vi "Pusher_Client_PingPong.vi"(8 "ErrIn":errorcluster, 11 "Client in":refnum<class "Client.lvclass">) -> (0 "ErrOut":errorcluster, 3 "Client out":refnum<class "Client.lvclass">)   [LabVIEW 2009, in "Client.lvclass"]
uses:
  Client.lvclass
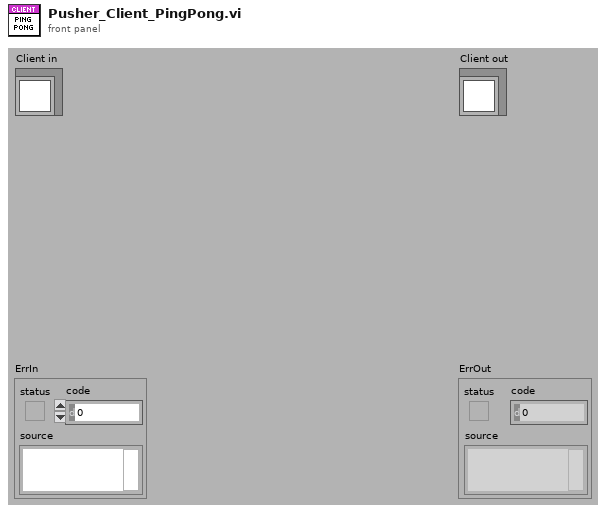
[diagram p1: front panel]
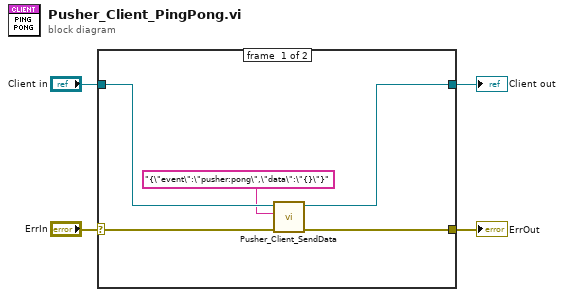
[diagram p0: block diagram]
diagram:
  n1 = case shown="No Error" "ErrIn" {
    selector: "ErrIn" -> [w9 w11]
    tunnel: [w8 w11] -> w3
    tunnel: [w6 w10] -> w1
    tunnel: "Client in" -> [w7 w10]
    frame #0 {
      n2 = call "Pusher_Client_SendData.vi"("ErrIn"=w9, "data"="{\"event\":\"pusher:pong\",\"data\":\"{}\"}", "Client in"=w7) -> ("ErrOut"=w8:errorcluster, "Client out"=w6:refnum<class "Client.lvclass">)  [unwired: 7 in]
    }
    frame #1 {
    }
  }
  "ErrOut" <- w3
  "Client out" <- w1
